vi "PWM3.vi"() -> ()   [LabVIEW 2019]
uses:
  <vilib>/rvi/Emulation/niFpgaGetClockAttributes.vi
  <vilib>/rvi/Emulation/niFpgaSctlEmulationGetInTimedLoop.vi
  <vilib>/rvi/Emulation/niFpgaEmulationReportErrorSimple.vi
  <vilib>/rvi/eio/common/nirviEmuTemplateMethod_errors.vi
  <vilib>/rvi/Emulation/niFpgaCriticalErrorInLSC.vi
  <vilib>/eio/EIONode/EIONode.xnode
panel:
  out "x-1":u32
  out "波形图表":u32(graph)
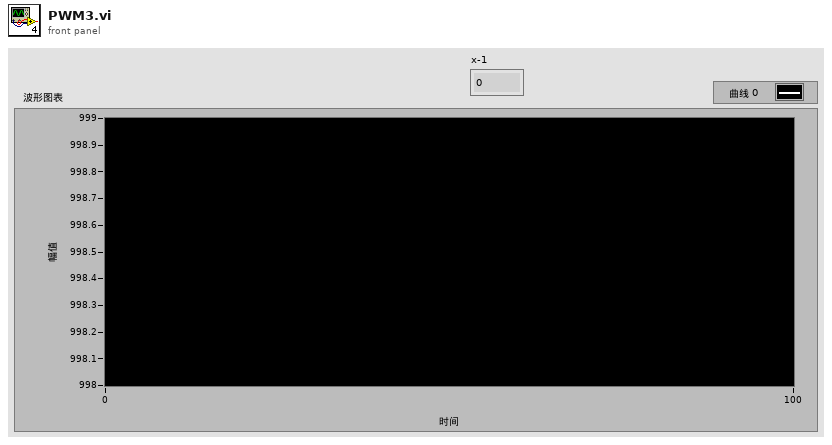
[diagram p1: front panel]
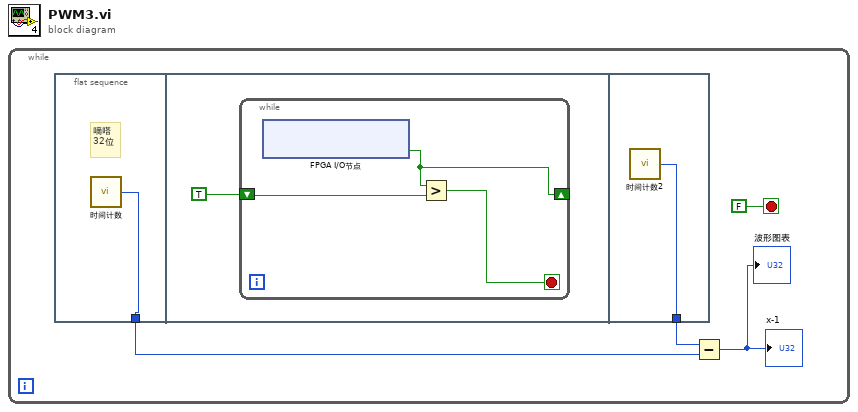
[diagram p0: block diagram]
diagram:
  n1 = while {
    stop <- FALSE stop-if-true
    n2 = flat-sequence {
      tunnel: [w5] -> w2
      tunnel: [w10] -> w3
      frame #0 {
        # "嘀嗒\n32位"
        n3 = call "时间计数"() -> ("Tick Count(Ticks)"=w5:u32)
      }
      frame #1 {
        n4 = while {
          shift-right: [w8] -> _
          shift-left: TRUE -> [w9]
          stop <- w7 stop-if-true
          n5 = xnode "FPGA I/O节点"() -> ("ConnectorB/DIO0"=w8:bool)  [unwired: 1 in, 1 out]
          n6 = Greater?(x=w8, y=w9) -> (0:w7:bool)
        }
      }
      frame #2 {
        n7 = call "时间计数2"() -> ("Tick Count(Ticks)"=w10:u32)
      }
    }
    n8 = Subtract(x=w3, y=w2) -> (x-y=→"x-1" →"波形图表":u32)
  }
